vi "draw_overlays.vi"(8 "error in (no error)":errorcluster, 11 "DL090623TwoDAnalyser in":refnum<class "AnalyserDL090623TwoD.lvclass">) -> (0 "error out":errorcluster, 3 "DL090623TwoDAnalyser out":refnum<class "AnalyserDL090623TwoD.lvclass">)   [LabVIEW 2010, in "AnalyserDL090623TwoD.lvclass"]
uses:
  AnalyserDL090623TwoD.lvclass
  AnalyserDL090623TwoD.lvclass/AnalyserDL090623TwoD.ctl
  common/classes/Image/Image/Image.lvclass
  common/classes/ErrorController/ErrorController/class_data.vi
  common/classes/ErrorController/ErrorController/ErrorController.lvclass
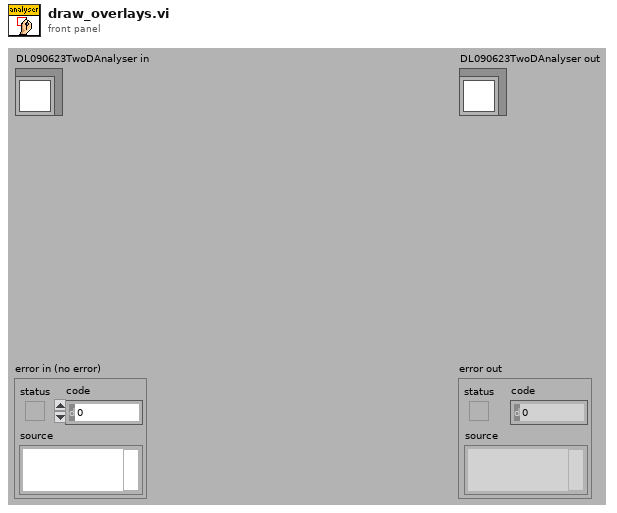
[diagram p1: front panel]
types:
  T1 = typedef "ROI Descriptor" = cluster{"Global Rectangle":i32[], "Contours":cluster{"ID":enum32{"External", "Internal"}, "Type":u32, "Coordinates":i32[]}[]}
  T2 = typedef "IMAQ Image.ctl" = refnum<image>
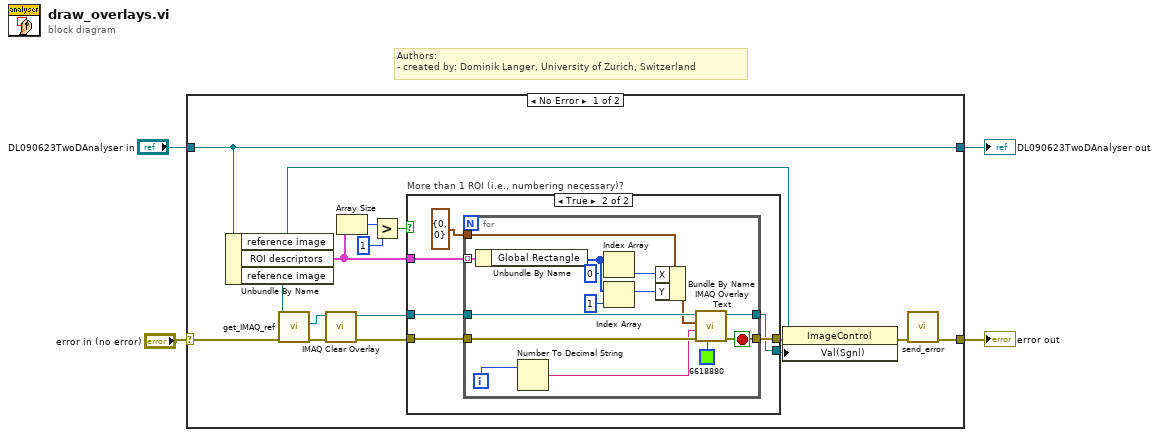
[diagram p0: block diagram]
diagram:
  # "Authors: \n- created by: Dominik Langer, University of Zurich, Switzerland"
  n1 = case shown="No Error" "error in (no error)" {
    selector: "error in (no error)" -> [w19 w45]
    tunnel: [w5 w45] -> w3
    tunnel: [w14 w44] -> w1
    tunnel: "DL090623TwoDAnalyser in" -> [w14 w44]
    frame No Error {
      n2 = Unbundle By Name(w14) -> ("reference image"=w13:refnum<vi>, "ROI descriptors"=w10:T1[], "reference image"=w20:refnum<class "Image.lvclass">)
      n3 = call-dynamic "get_IMAQ_ref.vi"("error in (no error)"=w19, "Image.lvclass in"=w20) -> ("error out"=w18:errorcluster, "Image"=w17:T2)  [unwired: 8 out]
      n4 = call "IMAQ Clear Overlay"("error in (no error)"=w18, "Image"=w17) -> ("error out"=w16:errorcluster, "Image Out"=w15:T2)  [unwired: 1 in, 7 out]
      n5 = Array Size(array=w10) -> (size(s)=w9:i32)
      n6 = Greater?(x=w9, y=1) -> (0:w7:bool)
      n7 = case "More than 1 ROI (i.e., numbering necessary)?" shown="True" w7 {
        tunnel: w10 -> [_ w28]
        tunnel: w16 -> [w22 w27]
        tunnel: w15 -> [w21 w26]
        tunnel: [w22 w24] -> w12
        tunnel: [w21 w23] -> w11
        frame False {
        }
        frame True {
          n8 = for {
            tunnel: w28 -> [w41] mode=indexing
            tunnel: w26 -> [w42]
            tunnel: cluster{"X":i32, "Y":i32} {"X"=0, "Y"=0} ("Origin") -> [w37]
            tunnel: [w30] -> w23
            tunnel: w27 -> [w43]
            tunnel: [w29] -> w24
            i -> [w33]
            stop <- w29 stop-if-true
            n9 = Unbundle By Name(w41) -> ("Global Rectangle"=w40:i32[])
            n10 = Number To Decimal String(number=w33) -> (decimal integer string=w32:string)  [unwired: 1 out]
            n11 = Index Array(array=w40, index=0) -> (element=w36:i32)
            n12 = Index Array(array=w40, index=1) -> (element=w35:i32)
            n13 = Bundle By Name(cluster=w37, "X"=w36, "Y"=w35) -> (w34:cluster{"X":i32, "Y":i32})
            n14 = call "IMAQ Overlay Text"("Text Color (black)"=u32 6618880, "error in (no error)"=w43, "String"=w32, "Origin"=w34, "Image"=w42) -> ("error out"=w29:errorcluster, "Image Out"=w30:T2)  [unwired: 3 in, 2 out]
          }
        }
      }
      n15 = property class="ImageControl"(reference=w13, error in=w12, "Val(Sgnl)"=w11) -> (error out=w6:errorcluster)  [unwired: 1 out]
      n16 = call "send_error.vi"("error in (no error)"=w6) -> ("error out"=w5:errorcluster)  [unwired: 10 in]
    }
    frame Error {
    }
  }
  "error out" <- w3
  "DL090623TwoDAnalyser out" <- w1
